vi "Translate.vi"(8 "error in (no error)":errorcluster, 10 "Offset":cluster{"dx":sgl, "dy":sgl}, 11 "Canvas in":refnum<class "Drawer .Net.lvclass">) -> (0 "error out":errorcluster, 3 "Canvas out":refnum<class "Drawer .Net.lvclass">)   [LabVIEW 2023, in "Glyph .NET Drawer.lvlib" / "Drawer .Net.lvclass"]
uses:
  Drawer .Net.lvclass
  Drawer .Net.lvclass/Drawer .Net.ctl
  System.Drawing
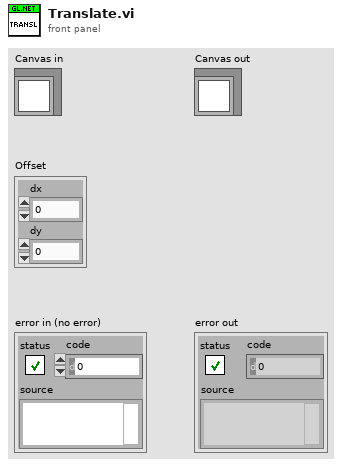
[diagram p1: front panel]
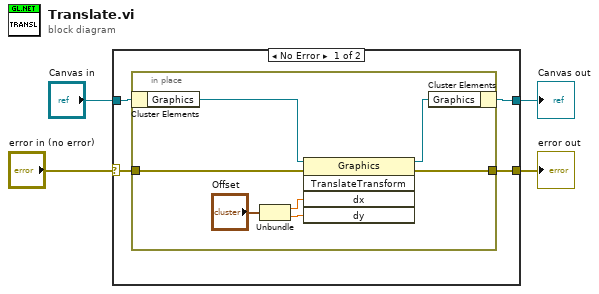
[diagram p0: block diagram]
diagram:
  n1 = case shown="No Error" "error in (no error)" {
    selector: "error in (no error)" -> [w6 w17]
    tunnel: [w5 w17] -> w3
    tunnel: [w7 w16] -> w1
    tunnel: "Canvas in" -> [w8 w16]
    frame No Error {
      n2 = in-place {
        in-place-border: w6 -> [w13]
        in-place-border: [w12] -> w5
        n3 = in-place-cluster #1(w8) -> ("Graphics"=w15:refnum<k24>)
        n4 = Unbundle("Offset") -> ("dx"=w11:sgl, "dy"=w10:sgl)
        n5 = invoke class="Graphics" method="TranslateTransform"(reference=w15, error in=w13, "dx"=w11, "dy"=w10) -> (reference out=w14:refnum<k24>, error out=w12:errorcluster)  [unwired: 1 in, 3 out]
        n6 = in-place-cluster #1("Graphics"=w14) -> (w7:refnum<class "Drawer .Net.lvclass">)
      }
    }
    frame Error {
    }
  }
  "error out" <- w3
  "Canvas out" <- w1
